vi "Obtain.vi"(8 "error in (no error)":errorcluster, 11 "Await interaction?(F)":bool) -> (0 "error out":errorcluster, 3 "Get Refnum out":refnum<class "Get Refnum.lvclass">)   [LabVIEW 2020, in "Msg.lvlib" / "Get Refnum.lvclass"]
doc: "Obtain a queue and populate the private data with the created queue."
uses:
  Get Refnum.lvclass
  Get Refnum.lvclass/Get Refnum.ctl
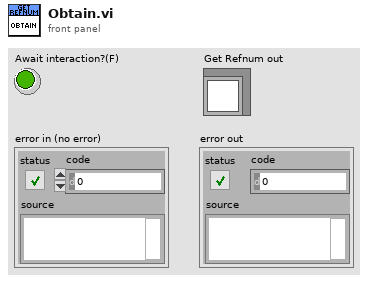
[diagram p1: front panel]
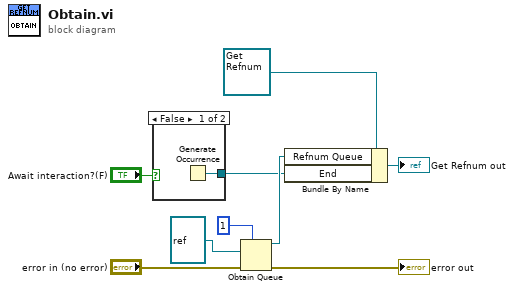
[diagram p0: block diagram]
diagram:
  n1 = case shown="False" "Await interaction?(F)" {
    tunnel: [w10 _] -> w2
    frame False {
      n2 = Generate Occurrence() -> (w10:refnum<k4>)
    }
    frame True {
    }
  }
  n3 = Obtain Queue(max queue size (-1, unlimited)=1, element data type=refnum<vi> refnum ("VI Refnum in"), error in (no error)="error in (no error)") -> (queue out=w6:refnum<queue>, error out=→"error out":errorcluster)  [unwired: 2 in, 1 out]
  n4 = Bundle By Name(cluster=refnum<class "Get Refnum.lvclass"> refnum ("Msg.lvlib:Display.lvclass"), "Refnum Queue"=w6, "End"=w2) -> (→"Get Refnum out":refnum<class "Get Refnum.lvclass">)
